vi "Motor_Banda_Transportadora.vi"() -> ()   [LabVIEW 2020]
panel:
  out "Motor Banda Transportadora":bool
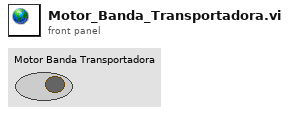
[diagram p1: front panel]
diagram:
